vi "Split String Around Character.vi"(9 "search string/char ( _ )":string="_", 10 "String in":string) -> (1 "String after":string, 2 "String before":string)   [LabVIEW 2021, in "Strings.lvlib"]
uses:
  Strings.lvlib
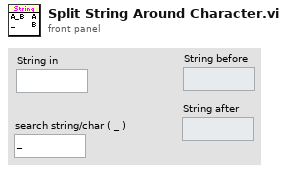
[diagram p1: front panel]
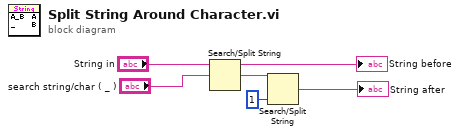
[diagram p0: block diagram]
diagram:
  n1 = Search/Split String(string="String in", search string/char (-)="search string/char ( _ )") -> (substring before match=→"String before":string, match + rest of string=w3:string)  [unwired: 1 in, 1 out]
  n2 = Search/Split String(string=w3, offset (0)=1) -> (match + rest of string=→"String after":string)  [unwired: 1 in, 2 out]
